vi "modify tag.vi"(4 "original tag name":string, 5 "Number of Elements":u32=1, 6 "original network path":string, 7 "eip tag types":T1, 8 "error in":errorcluster, 9 "Tag Name":string, 10 "Network Path":string, 11 "EIP Tags configuration in":refnum<class "EIP Tags Configuration.lvclass">) -> (0 "error out":errorcluster, 2 "removed channels":refnum<class "EIP Tags Channel.lvclass">[](array[class]), 3 "EIP Tags configuration out":refnum<class "EIP Tags Configuration.lvclass">)   [LabVIEW 2013, in "EIP Tags Configuration.lvclass"]
uses:
  EIP Tags Configuration.lvclass
  eip tag types.ctl
  channel/EIP Tags Channel.lvclass
  EIP Tags Configuration.lvclass/EIP Tags Configuration.ctl
  channel/EIP Tags Channel.lvclass/EIP Tags Channel.ctl
  <vilib>/NI/Tag Bus/tag/tag descriptor.lvclass/tag descriptor.ctl
  channel/Write EIP Tag UUID.vi
  <vilib>/NI/Tag Bus/tag/write data type.vi
  channel/Read element.vi
  channel/Read EIP Tag UUID.vi
  <vilib>/NI/Tag Bus Module Framework/root configuration/TBM configuration.lvclass
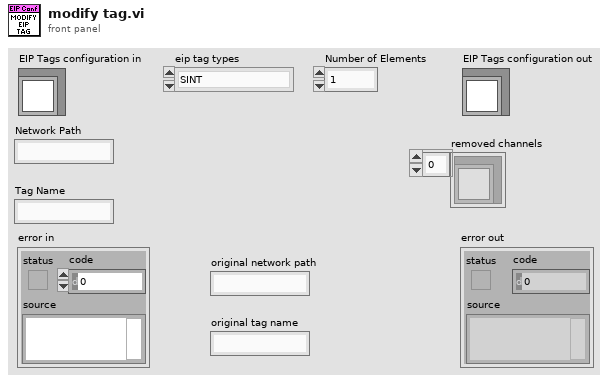
[diagram p1: front panel]
types:
  T1 = typedef "EIP Tags Configuration.lvclass/eip tag types.ctl" = enum16{"SINT", "INT", "DINT", "REAL", "BOOL", "STRING"}
  T2 = typedef "EIP Tags Configuration.lvclass/eip tag definition.ctl" = cluster{"eip tag types":T1, "unique tag name":string, "Number of Elements":u32}
  T3 = typedef "tag bus.lvlib/tag descriptor.lvclass/Data Type.ctl" = enum16{"Double", "Single", "I64", "I32", "I16", "I8", "U64", "U32", "U16", "U8", "Boolean", "String", "Array of Double", "Array of Single", "Array of I64", "Array of I32", "Array of I16", "Array of I8", "Array of U64", "Array of U32", "Array of U16", "Array of U8", "Array of Boolean", "Array of String"}
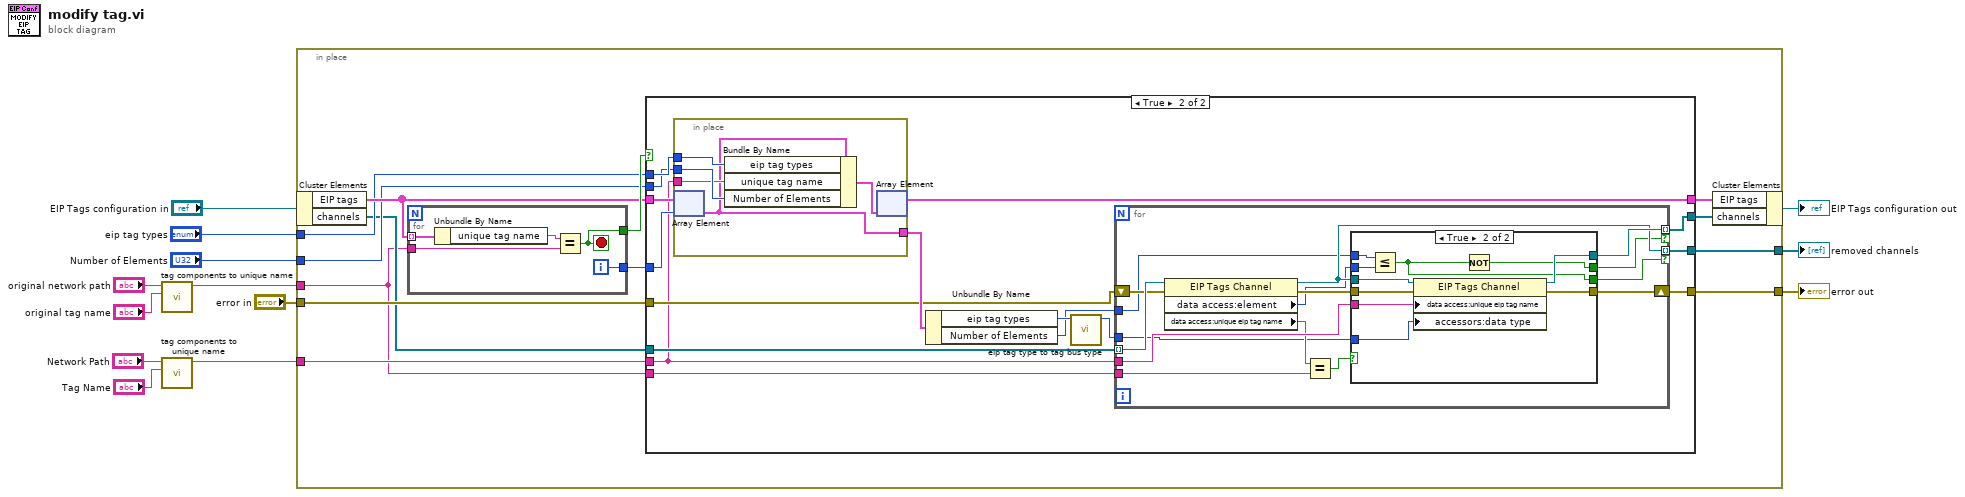
[diagram p0: block diagram]
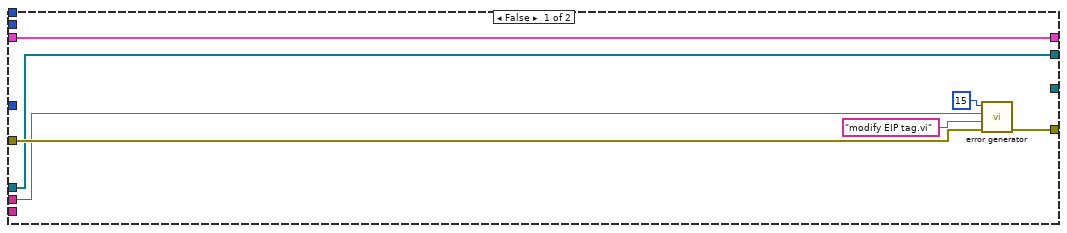
[diagram p2: hidden frame]
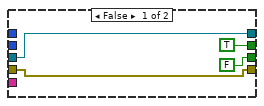
[diagram p3: hidden frame]
diagram:
  n1 = call "tag components to unique name.vi"("Tag Name"="original tag name", "Network Path"="original network path") -> ("unique name"=w2:string)  [unwired: 9 in]
  n2 = call "tag components to unique name.vi"("Tag Name"="Tag Name", "Network Path"="Network Path") -> ("unique name"=w8:string)  [unwired: 9 in]
  n3 = in-place {
    in-place-border: "error in" -> [w24]
    in-place-border: w8 -> [w21]
    in-place-border: [w25] -> w7
    in-place-border: "eip tag types" -> [w20]
    in-place-border: "Number of Elements" -> [w19]
    in-place-border: w2 -> [w15]
    in-place-border: [w14] -> w1
    n4 = in-place-cluster #1("EIP Tags configuration in") -> ("EIP tags"=w22:T2[], "channels"=w17:refnum<class "EIP Tags Channel.lvclass">[])
    n5 = for {
      tunnel: w22 -> [w88] mode=indexing
      tunnel: w15 -> [w86]
      tunnel: [w85] -> w26
      tunnel: [w84] -> w18
      i -> [w84]
      stop <- w85 stop-if-true
      n6 = Unbundle By Name(w88) -> ("unique tag name"=w87:string)
      n7 = Equal?(x=w87, y=w86) -> (x = y?=w85:bool)
    }
    n8 = case shown="True" w26 {
      tunnel: [w33 w39] -> w25
      tunnel: w24 -> [w32 w42]
      tunnel: [w30 w48] -> w23
      tunnel: w22 -> [w30 w49]
      tunnel: w21 -> [w29 w40]
      tunnel: w20 -> [_ w46]
      tunnel: w19 -> [_ w45]
      tunnel: w18 -> [_ w47]
      tunnel: w17 -> [w27 w43]
      tunnel: [w27 w38] -> w16
      tunnel: w15 -> [_ w41]
      tunnel: [_ w37] -> w14
      frame False {
        n9 = call <vilib>:"error generator.vi"("error in"=w32, "source"="modify EIP tag.vi", "append error message"=w29, "error code (0)"=15) -> ("error out"=w33:errorcluster)  [unwired: 7 in]
      }
      frame True {
        n10 = in-place {
          in-place-border: w46 -> [w82]
          in-place-border: w45 -> [w81]
          in-place-border: w40 -> [w80]
          in-place-border: [w79] -> w44
          n11 = in-place-array #2(w49, w47) -> (w79:T2)
          n12 = Bundle By Name(cluster=w79, "eip tag types"=w82, "unique tag name"=w80, "Number of Elements"=w81) -> (w83:T2)
          n13 = in-place-array #2(w83) -> (w48:T2[])  [unwired: 1 out]
        }
        n14 = Unbundle By Name(w44) -> ("eip tag types"=w36:T1, "Number of Elements"=w34:u32)
        n15 = call "eip tag type to tag bus type.vi"("eip tag types"=w36) -> ("data type"=w35:T3)  [unwired: 10 in]
        n16 = for {
          tunnel: w43 -> [w64] mode=indexing
          shift-right: [w61] -> w39
          shift-left: w42 -> [w63]
          tunnel: w41 -> [w60]
          tunnel: w40 -> [w58]
          tunnel: [w56] -> w38 mode=indexing if=w53
          tunnel: [w55] -> w37 mode=indexing if=w54
          tunnel: w35 -> [w51]
          tunnel: w34 -> [w50]
          n17 = property class="EIP Tags Channel"(reference=w64, error in=w63) -> (reference out=w55:refnum<class "EIP Tags Channel.lvclass">, error out=w62:errorcluster, "data access:element"=w52:i32, "data access:unique eip tag name"=w57:string)
          n18 = Equal?(x=w57, y=w60) -> (x = y?=w59:bool)
          n19 = case shown="True" w59 {
            tunnel: w55 -> [w68 w78]
            tunnel: w62 -> [w67 w77]
            tunnel: [w67 w76] -> w61
            tunnel: w58 -> [_ w75]
            tunnel: [w68 w74] -> w56
            tunnel: [FALSE w70] -> w54
            tunnel: [TRUE w69] -> w53
            tunnel: w52 -> [_ w71]
            tunnel: w51 -> [_ w73]
            tunnel: w50 -> [_ w72]
            frame False {
            }
            frame True {
              n20 = Less Or Equal?(x=w72, y=w71) -> (x <= y?=w70:bool)
              n21 = property class="EIP Tags Channel"(reference=w78, error in=w77, "data access:unique eip tag name"=w75, "accessors:data type"=w73) -> (reference out=w74:refnum<class "EIP Tags Channel.lvclass">, error out=w76:errorcluster)
              n22 = Not(x=w70) -> (.not. x?=w69:bool)
            }
          }
        }
      }
    }
    n23 = in-place-cluster #1("EIP tags"=w23, "channels"=w16) -> (→"EIP Tags configuration out":refnum<class "EIP Tags Configuration.lvclass">)
  }
  "error out" <- w7
  "removed channels" <- w1
